vi "To String.vi"(8 "error in (no error)":errorcluster, 11 "JSON Numeric in":refnum<class "JSON Numeric.lvclass">) -> (0 "error out":errorcluster, 3 "String":string)   [LabVIEW 2017, in "LVJSON.lvlib" / "JSON Numeric.lvclass"]
uses:
  JSON Numeric.lvclass
  JSON Numeric.lvclass/JSON Numeric.ctl
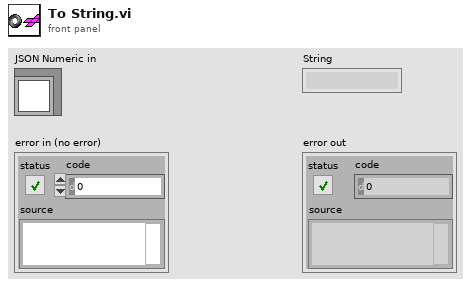
[diagram p1: front panel]
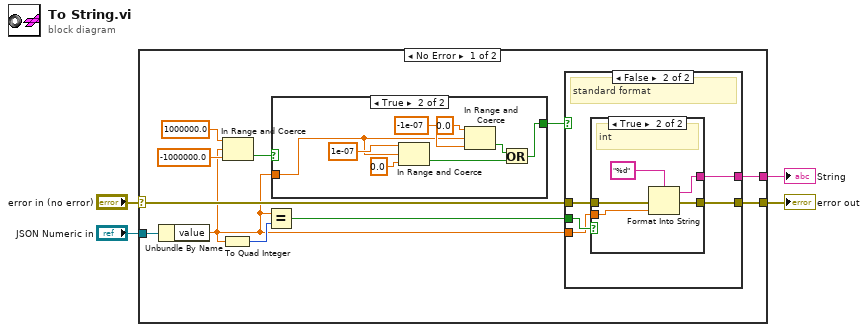
[diagram p0: block diagram]
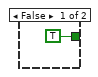
[diagram p2: hidden frame]
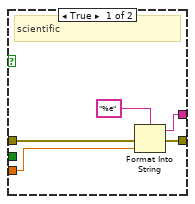
[diagram p3: hidden frame]
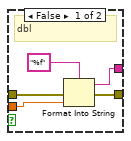
[diagram p4: hidden frame]
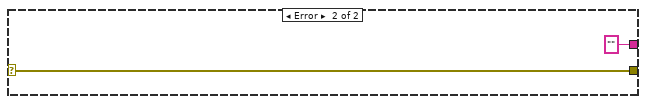
[diagram p5: hidden frame]
diagram:
  n1 = case shown="No Error" "error in (no error)" {
    selector: "error in (no error)" -> [w13 w46]
    tunnel: "JSON Numeric in" -> [w15 _]
    tunnel: [w12 ""] -> w2
    tunnel: [w11 w46] -> w1
    frame No Error {
      n2 = Unbundle By Name(w15) -> ("value"=w5:dbl)
      n3 = To Quad Integer(1:w5) -> (0:w10:i64)
      n4 = In Range and Coerce(upper limit=1000000.0, x=w5, lower limit=-1000000.0) -> (In Range?=w7:bool)  [unwired: 1 out]
      n5 = Equal?(x=w5, y=w10) -> (x = y?=w14:bool)
      n6 = case shown="True" w7 {
        tunnel: [TRUE w17] -> w6
        tunnel: w5 -> [_ w18]
        frame False {
        }
        frame True {
          n7 = In Range and Coerce(upper limit=1e-07, x=w18, lower limit=0.0) -> (In Range?=w24:bool)  [unwired: 1 out]
          n8 = In Range and Coerce(upper limit=0.0, x=w18, lower limit=-1e-07) -> (In Range?=w23:bool)  [unwired: 1 out]
          n9 = Or(x=w23, y=w24) -> (x .or. y?=w17:bool)
        }
      }
      n10 = case shown="False" w6 {
        tunnel: w14 -> [_ w34]
        tunnel: w13 -> [w29 w33]
        tunnel: w5 -> [w25 w32]
        tunnel: [w28 w31] -> w12
        tunnel: [w27 w30] -> w11
        frame True {
          # "scientific"
          n11 = Format Into String(format string="%e", error in=w29, w25) -> (resulting string=w28:string, error out=w27:errorcluster)  [unwired: 1 in]
        }
        frame False {
          # "standard format"
          n12 = case shown="True" w34 {
            tunnel: w33 -> [w36 w42]
            tunnel: w32 -> [w39 w40]
            tunnel: [w37 w43] -> w31
            tunnel: [w35 w41] -> w30
            frame False {
              # "dbl"
              n13 = Format Into String(format string="%f", error in=w36, w39) -> (resulting string=w37:string, error out=w35:errorcluster)  [unwired: 1 in]
            }
            frame True {
              # "int"
              n14 = Format Into String(format string="%d", error in=w42, w40) -> (resulting string=w43:string, error out=w41:errorcluster)  [unwired: 1 in]
            }
          }
        }
      }
    }
    frame Error {
    }
  }
  "String" <- w2
  "error out" <- w1
